vi "Actor Core.vi"(8 "error in":errorcluster, 11 "Nested in":refnum<class "Home.lvclass">) -> (0 "error out":errorcluster, 3 "Actor out":refnum<class "Actor.lvclass">)   [LabVIEW 2024, in "Home.lvlib" / "Home.lvclass"]
doc: "(<B>Filename</B>: Actor Framework.lvlib:Actor.lvclass:Actor Core.vi)\n\nReceives messages to the actor, reacts to them, and initiates any error handling that may shut the actor down.\n\nDescendant classes may override this VI to append parallel tasks for the actor to complete while it handles messages. Overrides use the Call Parent Method node."
uses:
  Home.lvclass
  Home.lvclass/Home.ctl
  <vilib>/MGI/Panel Manager/Panel Actor/Panel Actor/Panel Actor.lvclass
  <vilib>/ActorFramework/Actor/Actor.lvclass
  Interactor Messages/Discover Nodes Msg/Discover Nodes Msg.lvclass
  Interactor Messages/Set Slave Node-ID Msg/Set Slave Node-ID Msg.lvclass
  Interactor Messages/Connect Msg/Connect Msg.lvclass
  Interactor Messages/Load EDS Msg/Load EDS Msg.lvclass
  C:/Program Files/National Instruments/LabVIEW 2025/vi.lib/MGI/Panel Manager/Panel Actor/Panel Actor/Panel Actor.lvclass
  C:/Program Files/National Instruments/LabVIEW 2025/vi.lib/ActorFramework/Actor/Actor.lvclass
  D:/git/CANopen-XNET/Example/Home/Home.lvclass
  Interactor Messages/Set CANopen Master Node-ID Msg/Set CANopen Master Node-ID Msg.lvclass
panel:
  in  "Node-ID":u8=127 format="0x%02x"
  in  "EDS Files":i32(listbox)
  out "EDS File Valid":bool
  in  "EDS File Path":path
  in  "Load EDS File":bool
  out "Slave Node Valid":bool
  in  "Node-ID":u8=1 format="%02x"
  out "Connected":bool
  in  "Baud Rate":u32(ring)=500000 items=["1000k"=1000000, "800k"=800000, "500k"=500000, "250k"=250000, "125k"=125000, "50k"=50000, "25k"=25000, "10k"=10000]
  in  "Select Node Button":bool
  in  "Communication Adapter Names":string(combo)
  in  "Connect Button":bool
  in  "Discover Nodes Button":bool
  in  "Nodes":i32(listbox)
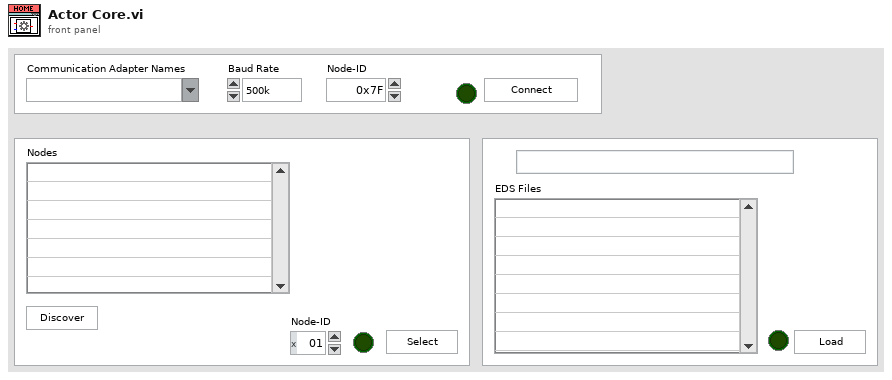
[diagram p1: front panel]
types:
  T1 = enum8{"Enabled", "Disabled", "Disabled and Grayed Out"}
  T2 = cluster{"Nodes List":refnum<user-event>, "Connected":refnum<user-event>, "Slave Node Selected":refnum<user-event>, "EDS File Valid":refnum<user-event>}
  T3 = cluster{"Event Registration Refnum":refnum<event-registration>, "Pnl Actor":refnum<event-registration>}
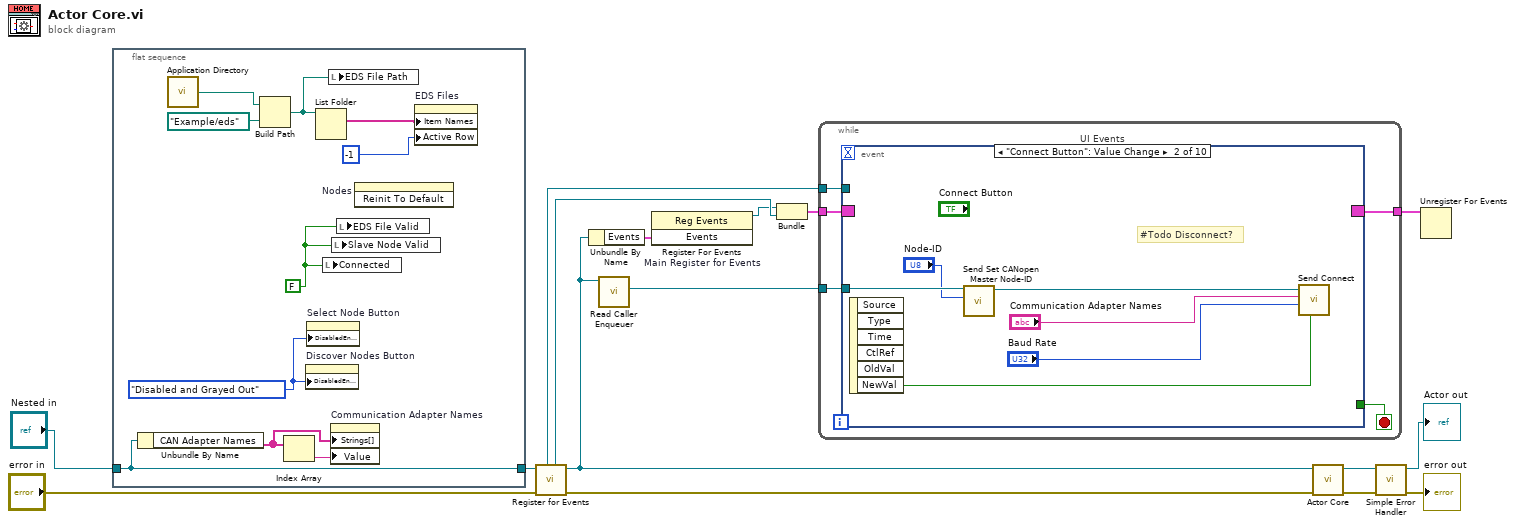
[diagram p0: block diagram]
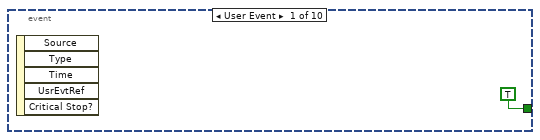
[diagram p2: hidden frame]
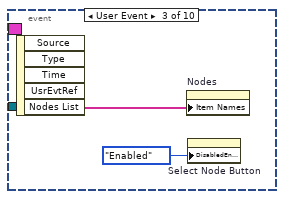
[diagram p3: hidden frame]
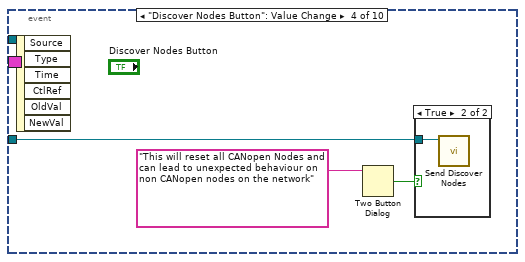
[diagram p4: hidden frame]
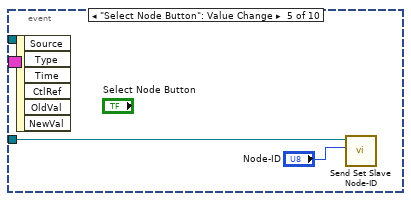
[diagram p6: hidden frame]
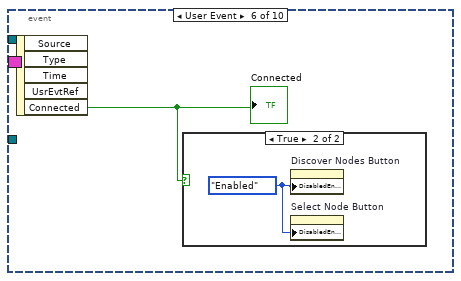
[diagram p7: hidden frame]
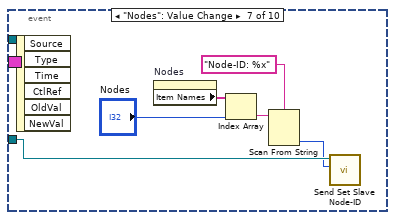
[diagram p9: hidden frame]
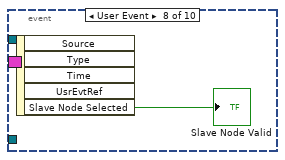
[diagram p10: hidden frame]
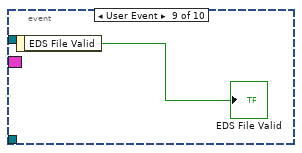
[diagram p11: hidden frame]
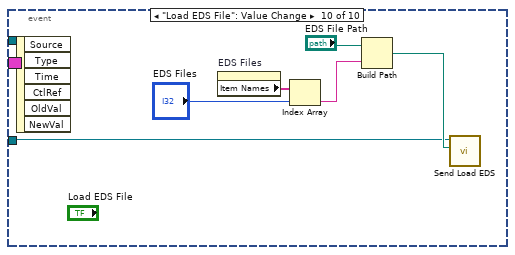
[diagram p12: hidden frame]
diagram:
  n1 = flat-sequence {
    tunnel: [w25] -> w7
    tunnel: "Nested in" -> [w25]
    frame #0 {
      w16 = FALSE ("Connect Button")
      w24 = T1."Disabled and Grayed Out" ("Disabled")
      n2 = Unbundle By Name(w25) -> ("CAN Adapter Names"=w22:string[])
      n3 = call <vilib>:"Application Directory.vi"() -> ("Application Directory"=w21:path)
      n4 = Build Path(base path=w21, name or relative path=path "Example/eds") -> (appended path=w19:path)
      n5 = Index Array(array=w22) -> (element=w23:string)  [unwired: 1 in]
      n6 = property on="Discover Nodes Button" class="Bool"("DisabledEnum"=w24) -> ()  [unwired: 2 in, 2 out]
      n7 = property on="Select Node Button" class="Bool"("DisabledEnum"=w24) -> ()  [unwired: 2 in, 2 out]
      n8 = List Folder(path=w19) -> (filenames=w18:string[])  [unwired: 3 in, 3 out]
      n9 = local write "Connected"(w16) -> ()
      n10 = local write "EDS File Path"(w19) -> ()
      n11 = property on="Communication Adapter Names" class="CmbBox"("Strings[]"=w22, "Value"=w23) -> ()  [unwired: 2 in, 2 out]
      n12 = local write "Slave Node Valid"(w16) -> ()
      n13 = local write "EDS File Valid"(w16) -> ()
      n14 = invoke on="Nodes" class="LstBox (strict)" method="Reinit To Default"() -> ()  [unwired: 3 in, 3 out]
      n15 = property on="EDS Files" class="LstBox (strict)"("Item Names"=w18, "Active Row"=-1 ("Active Row:Active Row Number")) -> ()  [unwired: 2 in, 2 out]
    }
  }
  n16 = call <vilib>:"Register for Events.vi"("Error In"="error in", "Panel Actor in"=w7) -> ("Error Out"=w8:errorcluster, "Panel Actor out"=w5:refnum<class "Home.lvclass">, "Pnl Actor"=w3:refnum<event-registration>, "Self Enqueuer"=w10:refnum<class "Message Enqueuer.lvclass">)  [unwired: 6 in]
  n17 = Unbundle By Name(w5) -> ("Events"=w13:T2)
  n18 = call <vilib>:"Read Caller Enqueuer.vi"("Actor"=w5) -> ("Caller Enqueuer"=w4:refnum<class "Message Enqueuer.lvclass">)  [unwired: 10 in]
  n19 = register-events "Main Register for Events"(w13) -> (reference out=w2:refnum<event-registration>)  [unwired: 2 in, 1 out]
  n20 = Bundle("Event Registration Refnum"=w2, "Pnl Actor"=w3) -> (w9:T3)  [unwired: 1 in]
  n21 = while {
    tunnel: w9 -> [w30]
    tunnel: [w28] -> w12
    tunnel: w10 -> [w27]
    tunnel: w4 -> [w26]
    stop <- w29 stop-if-true
    n22 = event "UI Events" shown="[1] \"Connect Button\": Value Change" {
      selector: w30 -> [_ _ _ _ _ _ _ _ _ _]
      dyn-events: [_ _ _ _ _ _ _ _ _ _] -> w28
      timeout: _ -> [_ _ _ _ _ _ _ _ _ _]
      tunnel: [TRUE _ _ _ _ _ _ _ _ _] -> w29
      tunnel: w27 -> [_ _ _ _ _ _ _ _ _ _]
      tunnel: w26 -> [_ w34 _ w42 w45 _ w49 _ _ w57]
      event User Event {
        n23 = event-data() -> ()  [unwired: 1 in, 5 out]
      }
      event "Connect Button": Value Change {
        # "#Todo Disconnect?"
        n24 = event-data() -> ("NewVal"=w35:bool)  [unwired: 1 in, 5 out]
        n25 = call "Send Set CANopen Master Node-ID.vi"("Node-ID"="Node-ID", "Message Enqueuer"=w34) -> ("Message Enqueuer out"=w32:refnum<class "Message Enqueuer.lvclass">)  [unwired: 8 in, 1 out]
        n26 = call "Send Connect.vi"("Connect/Disconnect"=w35, "Baud Rate"="Baud Rate", "ICommunicator Name"="Communication Adapter Names", "Message Enqueuer"=w32) -> ()  [unwired: 6 in, 2 out]
      }
      event User Event {
        n27 = event-data() -> ("Nodes List"=w39:string[])  [unwired: 1 in, 4 out]
        n28 = property on="Nodes" class="LstBox (strict)"("Item Names"=w39) -> ()  [unwired: 2 in, 2 out]
        n29 = property on="Select Node Button" class="Bool"("DisabledEnum"=T1."Enabled" ("Disabled")) -> ()  [unwired: 2 in, 2 out]
      }
      event "Discover Nodes Button": Value Change {
        n30 = event-data() -> ()  [unwired: 1 in, 6 out]
        n31 = Two Button Dialog(message="This will reset all CANopen Nodes and can lead to unexpected behaviour on non CANopen nodes on the network") -> (T button?=w41:bool)  [unwired: 2 in]
        n32 = case shown="True" w41 {
          tunnel: w42 -> [_ w43]
          frame False {
          }
          frame True {
            n33 = call "Send Discover Nodes.vi"("Message Enqueuer"=w43) -> ()  [unwired: 9 in, 2 out]
          }
        }
      }
      event "Select Node Button": Value Change {
        n34 = event-data() -> ()  [unwired: 1 in, 6 out]
        n35 = call "Send Set Slave Node-ID.vi"("Slave Node-ID"="Node-ID", "Message Enqueuer"=w45) -> ()  [unwired: 8 in, 2 out]
      }
      event User Event {
        n36 = event-data() -> ("Connected"=w46:bool)  [unwired: 1 in, 4 out]
        "Connected" <- w46
        n37 = case shown="True" w46 {
          frame False {
          }
          frame True {
            w47 = T1."Enabled" ("Disabled")
            n38 = property on="Discover Nodes Button" class="Bool"("DisabledEnum"=w47) -> ()  [unwired: 2 in, 2 out]
            n39 = property on="Select Node Button" class="Bool"("DisabledEnum"=w47) -> ()  [unwired: 2 in, 2 out]
          }
        }
      }
      event "Nodes": Value Change {
        n40 = event-data() -> ()  [unwired: 1 in, 6 out]
        n41 = property on="Nodes" class="LstBox (strict)"() -> ("Item Names"=w53:string[])  [unwired: 2 in, 2 out]
        n42 = Index Array(array=w53, index="Nodes") -> (element=w51:string)
        n43 = Scan From String(format string="Node-ID: %x", input string=w51) -> (output 1=w48:u8)  [unwired: 3 in, 3 out]
        n44 = call "Send Set Slave Node-ID.vi"("Slave Node-ID"=w48, "Message Enqueuer"=w49) -> ()  [unwired: 8 in, 2 out]
      }
      event User Event {
        n45 = event-data() -> ("Slave Node Selected"=→"Slave Node Valid":bool)  [unwired: 1 in, 4 out]
      }
      event User Event {
        n46 = event-data() -> ("EDS File Valid"=→"EDS File Valid":bool)  [unwired: 1 in]
      }
      event "Load EDS File": Value Change {
        n47 = event-data() -> ()  [unwired: 1 in, 6 out]
        n48 = property on="EDS Files" class="LstBox (strict)"() -> ("Item Names"=w60:string[])  [unwired: 2 in, 2 out]
        n49 = Index Array(array=w60, index="EDS Files") -> (element=w59:string)
        n50 = Build Path(base path="EDS File Path", name or relative path=w59) -> (appended path=w58:path)
        n51 = call "Send Load EDS.vi"("EDS File Path"=w58, "Message Enqueuer"=w57) -> ()  [unwired: 8 in, 2 out]
      }
    }
  }
  n52 = call-parent "Actor Core.vi"("error in"=w8, "Panel Actor in"=w5) -> ("error out"=w15:errorcluster, "Actor out"=→"Actor out":refnum<class "Actor.lvclass">)  [unwired: 8 in]
  n53 = call <vilib>:"Simple Error Handler.vi"("error in (no error)"=w15) -> ("error out"=→"error out":errorcluster)  [unwired: 4 in, 4 out]
  n54 = Unregister For Events(event registration refnum=w12) -> ()  [unwired: 1 in, 1 out]
